vi "Update Connection.vi"(8 "error in (no error)":errorcluster, 10 "TCP Data before update":T1, 11 "TCP Data after update":T1) -> (0 "error out":errorcluster, 3 "TCP Data after update out":T1)   [LabVIEW 2015, in "TCP.lvlib"]
uses:
  TCP.lvlib
  TypeDefs/TCP Data.ctl
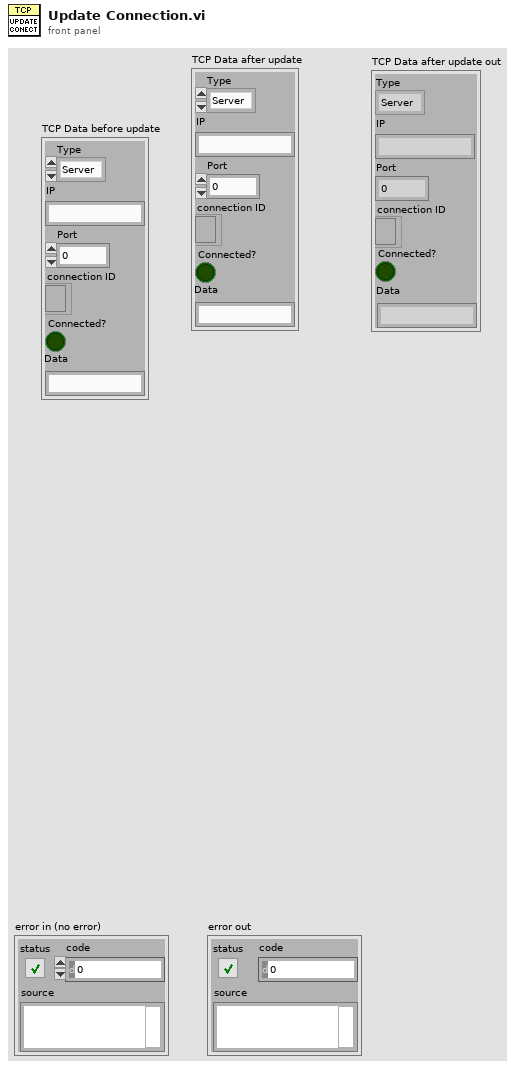
[diagram p1: front panel]
types:
  T1 = typedef "TCP.lvlib/TCP Data.ctl" = cluster{"Type":enum16{"Server", "Client"}, "IP":string, "Port":u16, "connection ID":refnum<k5>, "Connected?":bool, "Data":string}
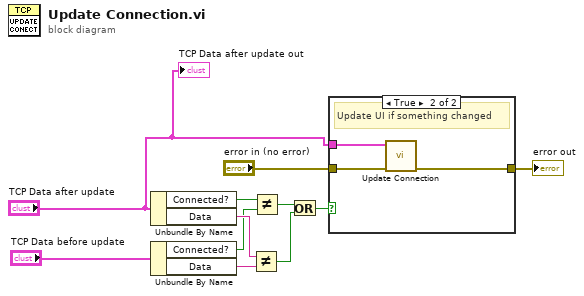
[diagram p0: block diagram]
diagram:
  n1 = Unbundle By Name("TCP Data after update") -> ("Connected?"=w4:bool, "Data"=w6:string)
  n2 = Unbundle By Name("TCP Data before update") -> ("Connected?"=w5:bool, "Data"=w7:string)
  n3 = Not Equal?(x=w6, y=w7) -> (x != y?=w9:bool)
  n4 = Not Equal?(x=w4, y=w5) -> (x != y?=w8:bool)
  n5 = Or(x=w8, y=w9) -> (x .or. y?=w10:bool)
  n6 = case shown="True" w10 {
    tunnel: "error in (no error)" -> [w12 w14]
    tunnel: [w12 w15] -> w11
    tunnel: "TCP Data after update" -> [_ w13]
    frame False {
    }
    frame True {
      # "Update UI if something changed"
      n7 = call "Update Connection.vi"("error in"=w14, "TCP Data"=w13) -> ("error out"=w15:errorcluster)  [unwired: 9 in]
    }
  }
  "error out" <- w11
  "TCP Data after update out" <- "TCP Data after update"
